vi "Autonomous Independent.vi"() -> ()   [LabVIEW 2014]
doc: "This VI is called when autonomous begins, and will automatically be terminated when autonomous ends. You can carry out timed or sensor driven robot movement independently without needing to return to the caller."
uses:
  <vilib>/Rock Robotics/WPI/DriverStation/WPI_DriverStationDerivedRobotMode.ctl
  <vilib>/Rock Robotics/WPI/DriverStation/WPI_DriverStationMatch Info.ctl
  <vilib>/Utility/file.llb/Read From Spreadsheet File (DBL).vi
  Global Variables.vi
panel:
  in  "Match Info":T1={"Autonomous Elapsed Seconds"=0.0, "TeleOp Elapsed Seconds"=0.0, "Disabled Elapsed Seconds"=0.0, "Visited Autonomous"=FALSE, "Visited TeleOp"=FALSE, "Visited Disabled"=FALSE, "Autonomous Settings"={"Autonomous Style"=enum."Independent", "VI Refnum"=refnum}}
  in  "Call Context":T2
  # "Be sure to right-click and choose Data Operations>>Make Current Value default if you want to save the array values with the VI"
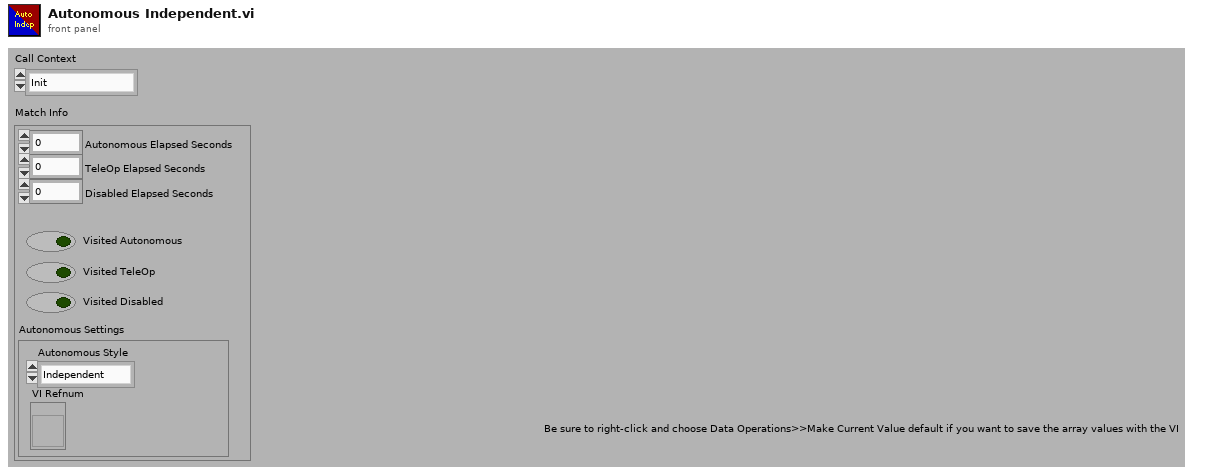
[diagram p1: front panel]
types:
  T1 = typedef "WPI_DriverStationMatch Info.ctl" = cluster{"Autonomous Elapsed Seconds":dbl, "TeleOp Elapsed Seconds":dbl, "Disabled Elapsed Seconds":dbl, "Visited Autonomous":bool, "Visited TeleOp":bool, "Visited Disabled":bool, "Autonomous Settings":cluster{"Autonomous Style":enum16{"Iterative", "Independent"}, "VI Refnum":refnum<vi>}}
  T2 = typedef "WPI_DriverStationDerivedRobotMode.ctl" = enum16{"Init", "Execute", "Stop"}
  T3 = typedef "WPI_JoystickDevRef.ctl" = cluster{"Device":T4}
  T4 = typedef "WPI_JoystickDeviceEnum.ctl" = enum16{"USB 0", "USB 1", "USB 2", "USB 3", "USB 4", "USB 5"}
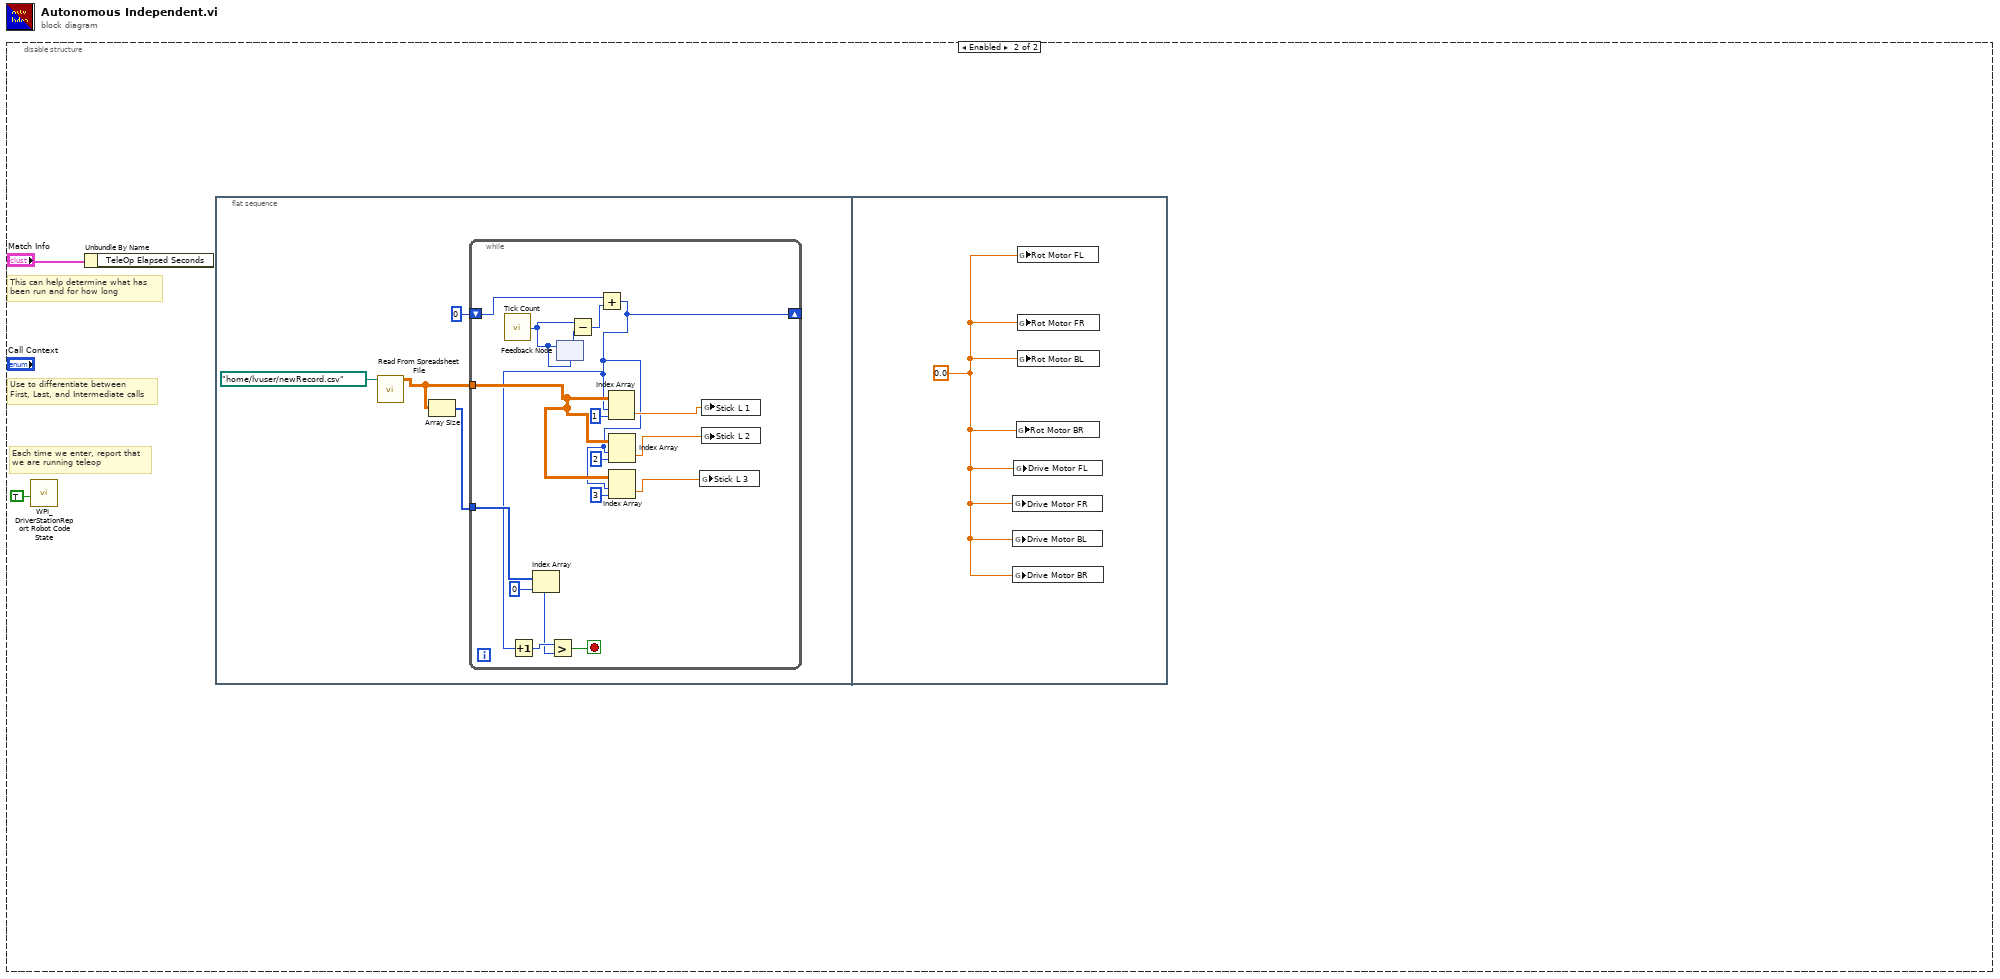
[diagram p0: block diagram]
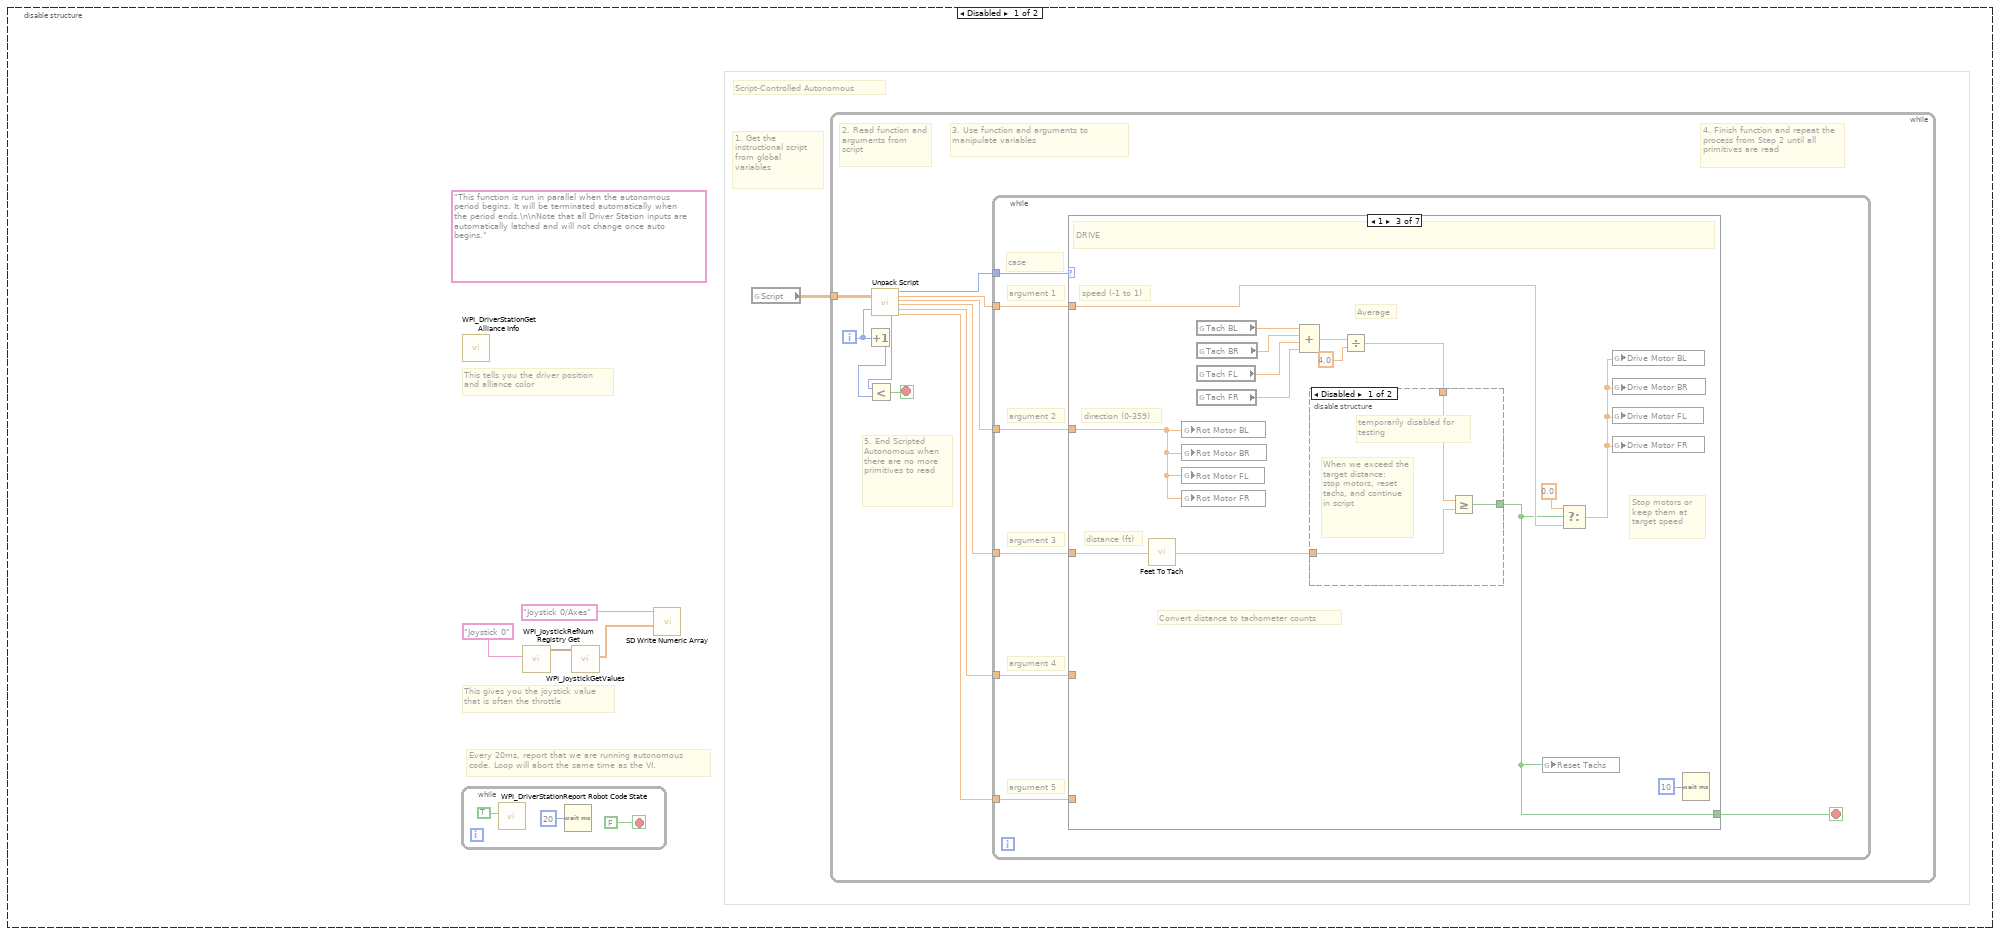
[diagram p2: hidden frame]
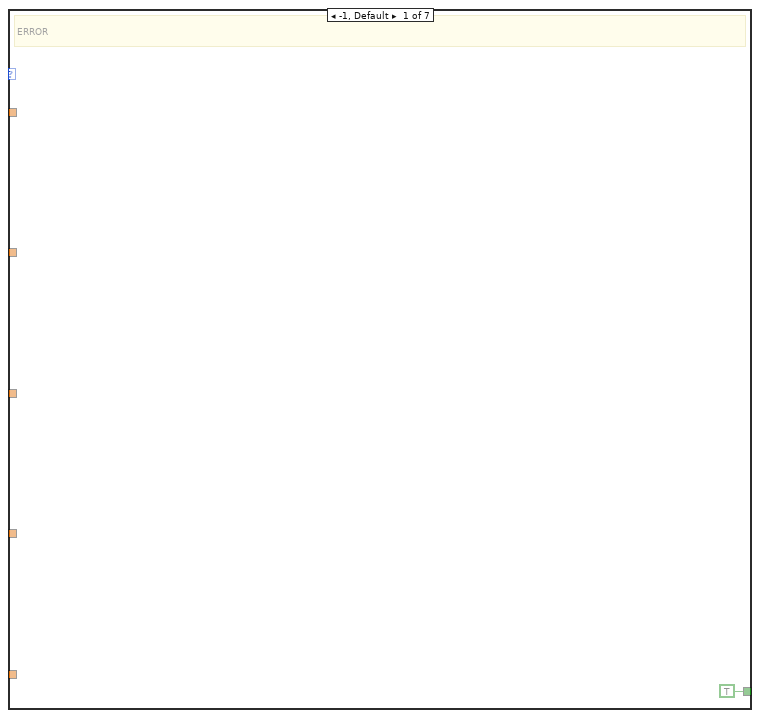
[diagram p3: hidden frame]
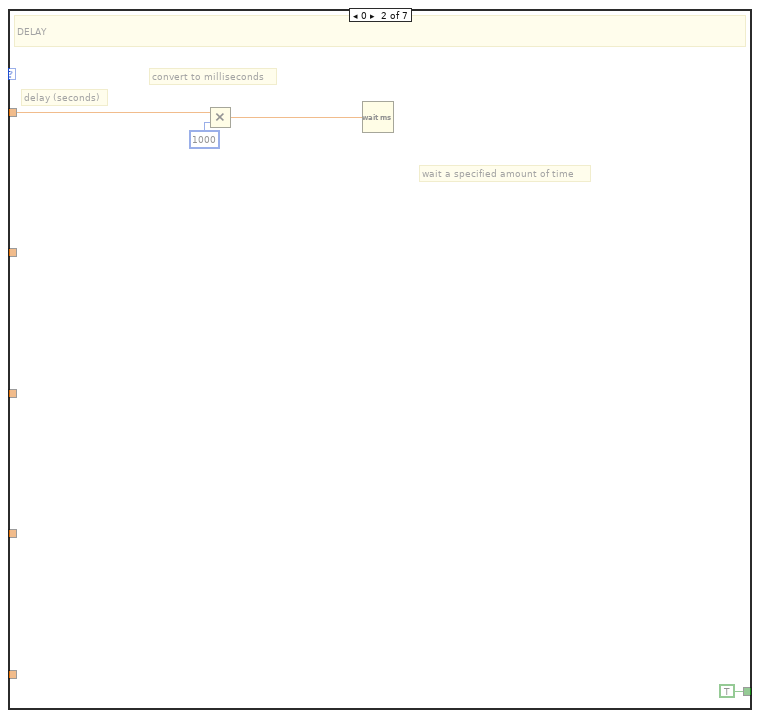
[diagram p4: hidden frame]
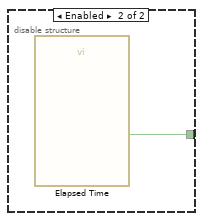
[diagram p5: hidden frame]
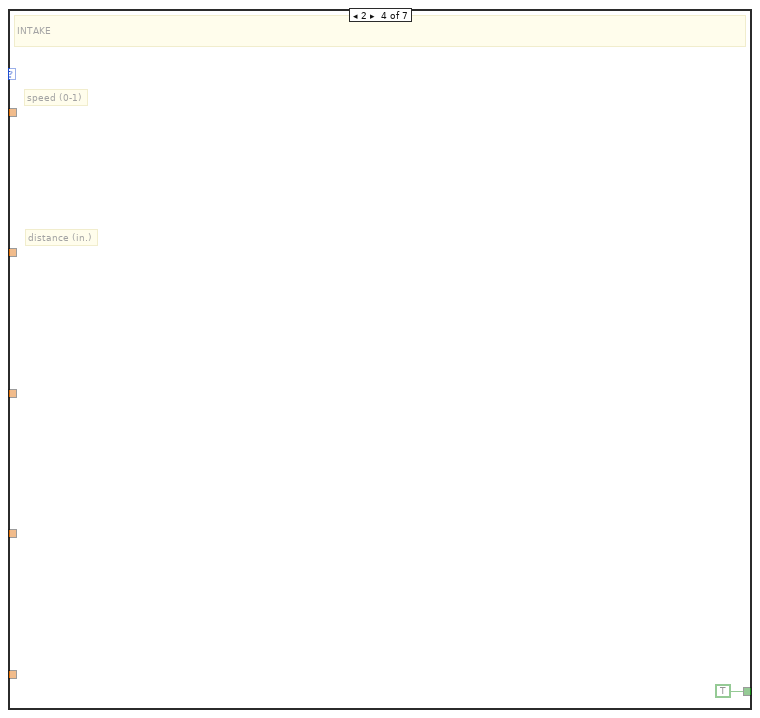
[diagram p6: hidden frame]
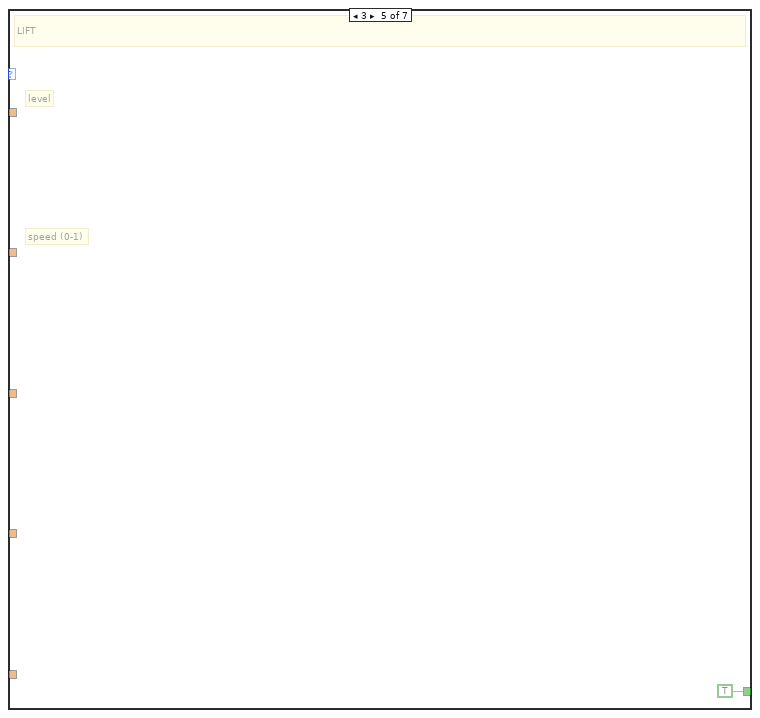
[diagram p7: hidden frame]
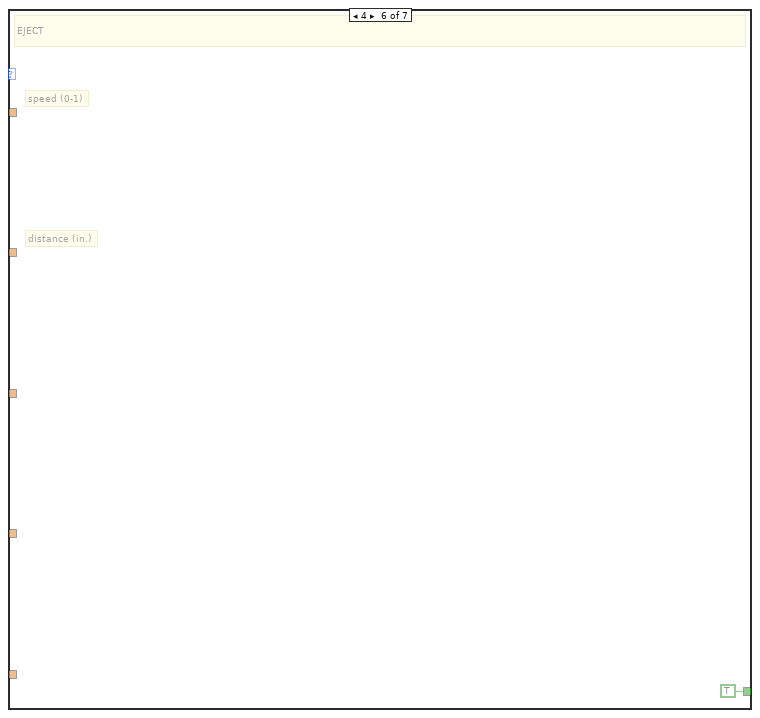
[diagram p8: hidden frame]
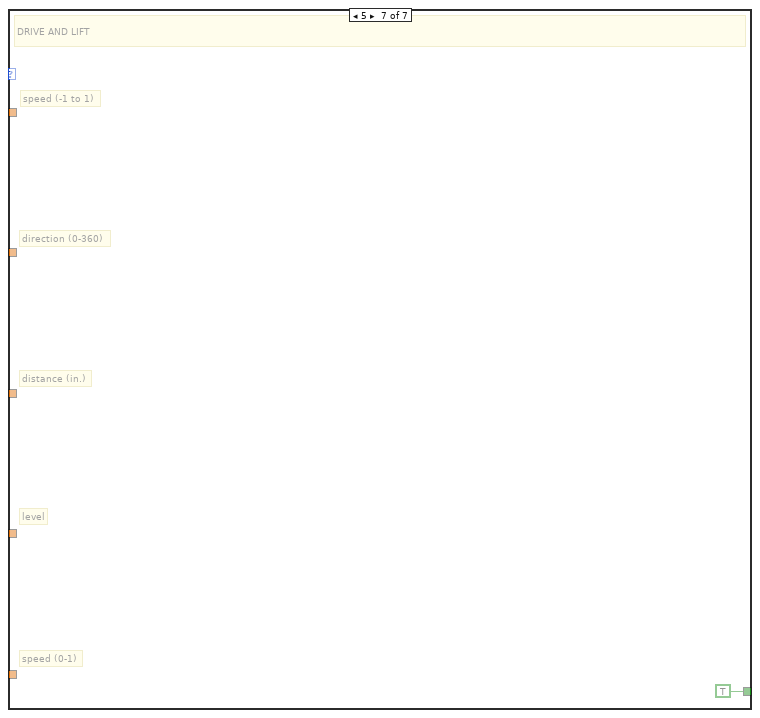
[diagram p9: hidden frame]
diagram:
  n1 = disable-structure shown="Enabled" {
    frame Disabled {
      (unwired) "This function is run in parallel when the autonomous period begins. It will be terminated automatically when the period ends.\n\nNote that all Driver Station inputs are automatically latched and will not change once auto begins."
      # "1. Get the instructional script from global variables"
      # "Script-Controlled Autonomous"
      # "Every 20ms, report that we are running autonomous\ncode. Loop will abort the same time as the VI."
      # "This gives you the joystick value\nthat is often the throttle"
      # "This tells you the driver position\nand alliance color"
      n2 = while {
        stop <- FALSE stop-if-true
        n3 = call <vilib>:"WPI_DriverStationReport Robot Code State.vi"("Autonomous"=TRUE) -> ()  [unwired: 10 in, 1 out]
        n4 = Wait (ms)(milliseconds to wait=u32 20) -> ()  [unwired: 1 out]
      }
      n5 = call <vilib>:"WPI_DriverStationGet Alliance Info.vi"() -> ()  [unwired: 12 out]
      n6 = call <vilib>:"WPI_JoystickRefNum Registry Get.vi"("refnum name"="Joystick 0") -> ("JoystickDevRef"=w4:T3)  [unwired: 1 in, 9 out]
      n7 = call <vilib>:"WPI_JoystickGetValues.vi"("JoystickDevRef"=w4) -> ("Axes"=w2:dbl[])  [unwired: 6 in, 4 out]
      n8 = call <vilib>:"SD Write Numeric Array.vi"("Numeric Array"=w2, "Name"="Joystick 0/Axes") -> ()  [unwired: 8 in, 2 out]
      n9 = global read "Global Variables.vi" "Script"() -> (w1:dbl[][])
      n10 = while {
        tunnel: w1 -> [w6]
        i -> [w10]
        stop <- w16 stop-if-true
        # "4. Finish function and repeat the process from Step 2 until all primitives are read"
        # "3. Use function and arguments to manipulate variables"
        # "5. End Scripted Autonomous when there are no more primitives to read"
        # "2. Read function and arguments from script"
        n11 = Increment(x=w10) -> (x+1=w8:i32)
        n12 = call "Unpack Script.vi"("script"=w6, "index"=w10) -> ("# of primitives"=w7:i32, "primitive"=w9:i32, "argument 1"=w15:dbl, "argument 2"=w14:dbl, "argument 3"=w13:dbl, "argument 4"=w12:dbl, "argument 5"=w11:dbl)  [unwired: 11 in]
        n13 = Less?(x=w7, y=w8) -> (x < y?=w16:bool)
        n14 = while {
          tunnel: w15 -> [w23]
          tunnel: w14 -> [w22]
          tunnel: w13 -> [w21]
          tunnel: w12 -> [w20]
          tunnel: w11 -> [w19]
          tunnel: w9 -> [w18]
          stop <- w17 stop-if-true
          # "case"
          # "argument 5"
          # "argument 4"
          # "argument 3"
          # "argument 2"
          # "argument 1"
          n15 = case shown="1" w18 {
            tunnel: w23 -> [_ w27 w34 _ _ _ _]
            tunnel: w22 -> [_ _ w31 _ _ _ _]
            tunnel: w21 -> [_ _ w43 _ _ _ _]
            tunnel: w20 -> [_ _ _ _ _ _ _]
            tunnel: w19 -> [_ _ _ _ _ _ _]
            tunnel: [TRUE TRUE w29 TRUE TRUE TRUE TRUE] -> w17
            frame -1, Default {
              # "ERROR"
            }
            frame 0 {
              # "wait a specified amount of time"
              # "convert to milliseconds"
              # "delay (seconds)"
              # "DELAY"
              n16 = Multiply(x=w27, y=1000) -> (x*y=w26:dbl)
              n17 = Wait (ms)(milliseconds to wait=w26) -> ()  [unwired: 1 out]
            }
            frame 1 {
              # "Stop motors or keep them at target speed"
              # "Average"
              # "Convert distance to tachometer counts"
              # "distance (ft)"
              # "direction (0-359)"
              # "speed (-1 to 1)"
              # "DRIVE"
              n18 = call "Feet To Tach.vi"("Feet"=w43) -> ("Tach Counts"=w35:dbl)
              n19 = global write "Global Variables.vi" "Rot Motor BL"(w31) -> ()
              n20 = global write "Global Variables.vi" "Rot Motor BR"(w31) -> ()
              n21 = global write "Global Variables.vi" "Rot Motor FL"(w31) -> ()
              n22 = global write "Global Variables.vi" "Rot Motor FR"(w31) -> ()
              n23 = global read "Global Variables.vi" "Tach BL"() -> (w42:dbl)
              n24 = global read "Global Variables.vi" "Tach BR"() -> (w41:dbl)
              n25 = global read "Global Variables.vi" "Tach FL"() -> (w40:dbl)
              n26 = global read "Global Variables.vi" "Tach FR"() -> (w39:dbl)
              n27 = Compound Arithmetic op=ADD(w42, w41, w40, w39) -> (w38:dbl)
              n28 = Divide(x=w38, y=4.0) -> (x/y=w36:dbl)
              n29 = disable-structure shown="Disabled" {
                disable-tunnel: w36 -> [w46 _]
                disable-tunnel: w35 -> [w45 _]
                disable-tunnel: [w44 w47] -> w29
                frame Disabled {
                  # "When we exceed the target distance: stop motors, reset tachs, and continue in script"
                  # "temporarily disabled for\ntesting"
                  n30 = Greater Or Equal?(x=w46, y=w45) -> (x >= y?=w44:bool)
                }
                frame Enabled {
                  n31 = call "Elapsed Time"() -> ("Time has Elapsed"=w47:bool)  [unwired: 12 in, 7 out]
                }
              }
              n32 = global write "Global Variables.vi" "Reset Tachs"(w29) -> ()
              n33 = Select(t=0.0, s=w29, f=w34) -> (s? t:f=w32:dbl)
              n34 = global write "Global Variables.vi" "Drive Motor BL"(w32) -> ()
              n35 = global write "Global Variables.vi" "Drive Motor BR"(w32) -> ()
              n36 = global write "Global Variables.vi" "Drive Motor FL"(w32) -> ()
              n37 = global write "Global Variables.vi" "Drive Motor FR"(w32) -> ()
              n38 = Wait (ms)(milliseconds to wait=u32 10) -> ()  [unwired: 1 out]
            }
            frame 2 {
              # "distance (in.)"
              # "speed (0-1)"
              # "INTAKE"
            }
            frame 3 {
              # "speed (0-1)"
              # "level"
              # "LIFT"
            }
            frame 4 {
              # "distance (in.)"
              # "speed (0-1)"
              # "EJECT"
            }
            frame 5 {
              # "speed (0-1)"
              # "level"
              # "distance (in.)"
              # "direction (0-360)"
              # "speed (-1 to 1)"
              # "DRIVE AND LIFT"
            }
          }
        }
      }
    }
    frame Enabled {
      # "Each time we enter, report that\nwe are running teleop"
      # "Use to differentiate between\nFirst, Last, and Intermediate calls"
      # "This can help determine what has\nbeen run and for how long"
      n39 = call <vilib>:"WPI_DriverStationReport Robot Code State.vi"("TeleOp"=TRUE ("Autonomous")) -> ()  [unwired: 10 in, 1 out]
      n40 = Unbundle By Name("Match Info") -> ()  [unwired: 1 out]
      n41 = flat-sequence {
        frame #0 {
          n42 = call-poly <vilib>:"Read From Spreadsheet File.vi"("file path (dialog if empty)"=path "/home/lvuser/newRecord.csv") -> ("all rows"=w59:dbl[][])  [unwired: 6 in, 4 out]
          n43 = Array Size(array=w59) -> (size(s)=w60:i32[])
          n44 = while {
            tunnel: w59 -> [w66]
            tunnel: w60 -> [w73]
            shift-right: [w61] -> _
            shift-left: u32 0 -> [w67]
            stop <- w62 stop-if-true
            n45 = call "Tick Count"() -> ("Tick Count(mSec)"=w69:u32)
            n46 = Index Array(array=w73, index=0) -> (element=w71:i32)
            n47 = feedback-in #1(w69) -> ()
            n48 = feedback #1(w69) -> (w70:u32)
            n49 = Subtract(x=w69, y=w70) -> (x-y=w68:u32)
            n50 = Add(x=w67, y=w68) -> (x+y=w61:u32)
            n51 = Increment(x=w61) -> (x+1=w74:u32)
            n52 = Greater?(x=w74, y=w71) -> (0:w62:bool)
            n53 = Index Array(array=w66, index (row)=w61, index (col)=1 ("disabled index (col)")) -> (element=w63:dbl)
            n54 = Index Array(array=w66, index (row)=w61, index (col)=2) -> (element=w64:dbl)
            n55 = Index Array(array=w66, index (row)=w61, index (col)=3) -> (element=w65:dbl)
            n56 = global write "Global Variables.vi" "Stick L 3"(w65) -> ()
            n57 = global write "Global Variables.vi" "Stick L 1"(w63) -> ()
            n58 = global write "Global Variables.vi" "Stick L 2"(w64) -> ()
          }
        }
        frame #1 {
          w78 = 0.0
          n59 = global write "Global Variables.vi" "Drive Motor FR"(w78) -> ()
          n60 = global write "Global Variables.vi" "Drive Motor BL"(w78) -> ()
          n61 = global write "Global Variables.vi" "Drive Motor BR"(w78) -> ()
          n62 = global write "Global Variables.vi" "Drive Motor FL"(w78) -> ()
          n63 = global write "Global Variables.vi" "Rot Motor BR"(w78) -> ()
          n64 = global write "Global Variables.vi" "Rot Motor FL"(w78) -> ()
          n65 = global write "Global Variables.vi" "Rot Motor FR"(w78) -> ()
          n66 = global write "Global Variables.vi" "Rot Motor BL"(w78) -> ()
        }
      }
    }
  }
